vi "build compound filter.vi"(7 "Type (OR)":enum16{"AND", "OR"}(ring)=enum."OR", 8 "error in (no error)":errorcluster, 9 "Filter B":refnum<k24>, 10 "Filter A":refnum<k24>, 11 "alias-tree in":refnum<class "alias-tree.lvclass">) -> (0 "error out":errorcluster, 2 "Compound Filter":refnum<k24>, 3 "alias-tree out":refnum<class "alias-tree.lvclass">)   [LabVIEW 2017, in "vs-tree-utility.lvlib" / "alias-tree.lvclass"]
uses:
  alias-tree.lvclass
  NationalInstruments.VeriStand.SystemStorage
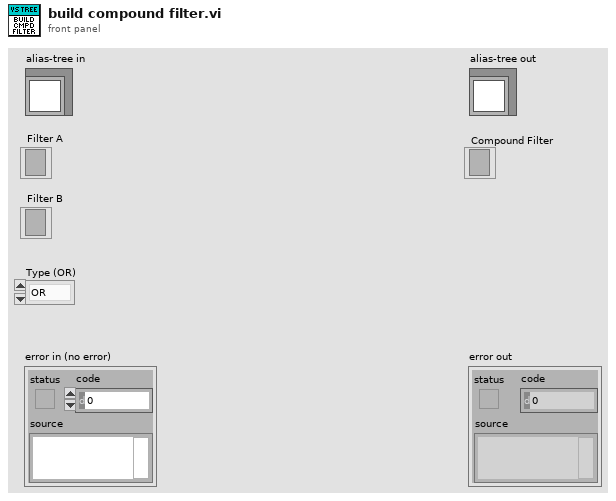
[diagram p1: front panel]
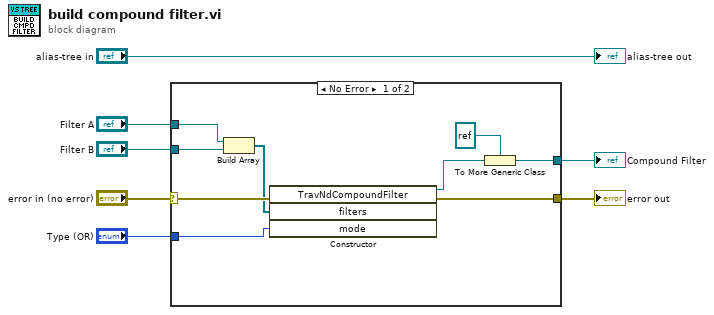
[diagram p0: block diagram]
diagram:
  n1 = case shown="No Error" "error in (no error)" {
    selector: "error in (no error)" -> [w16 w17]
    tunnel: [w15 w17] -> w6
    tunnel: "Type (OR)" -> [w14 _]
    tunnel: "Filter B" -> [w13 _]
    tunnel: "Filter A" -> [w12 _]
    tunnel: [w9 _] -> w2
    frame No Error {
      n2 = Build Array(w12, w13) -> (w11:refnum<k24>[])
      n3 = constructor class="TravNdCompoundFilter"(error in=w16, "filters"=w11, "mode"=w14) -> (reference out=w10:refnum<k24>, error out=w15:errorcluster)  [unwired: 2 in, 3 out]
      n4 = To More Generic Class(target class=refnum<k24> refnum ("customFilter"), reference=w10) -> (generic class reference=w9:refnum<k24>)
    }
    frame Error {
    }
  }
  "error out" <- w6
  "Compound Filter" <- w2
  "alias-tree out" <- "alias-tree in"
